vi "WAM_Datalog Parser.vi"() -> ()   [LabVIEW 2018]
uses:
  <vilib>/Utility/file.llb/Write Delimited Spreadsheet (DBL).vi
  <vilib>/Utility/file.llb/Read Delimited Spreadsheet (string).vi
  <vilib>/Utility/file.llb/Write Delimited Spreadsheet (string).vi
panel:
  out "Test Efficiency":string
  out "Fails Retested -Pass":i32
  out "Array":string[](array[string])
  out "pass_check-fails":string[](array[string])
  out "fails_check-pass":string[](array[string])
  out "Data 2":string[][](array[string])
  out "SN Search Result":string[][](array[string])
  in  "SN SEARCH":string
  out "tmp_path":path
  out "filenames":string[](array[string])
  out "Status":string
  out "Fails Repeated":i32
  out "Passes Repeated":i32
  out "#OfUnits_Adj":i32
  out "Total SN's Tested":i32
  out "#Passes_Adj":i32
  out "Pass Stats":cluster{"times":i32, "Word":string}[](array[cluster])
  out "Pass_sn":string[](array[string])
  out "Fails_Adj":i32
  out "No Of Words":i32
  out "Fail Stats":cluster{"times":i32, "Word":string}[](array[cluster])
  out "Fails_sn":string[](array[string])
  out "status":bool
  out "Message":string
  out "x > y?":bool
  in  "Get All Data(t)":bool
  out "Yield %":string
  out "Tested_Adj":i32
  out "End Date":string
  in  "Stop":timestamp
  out "Incompletes":string[][](array[string])
  out "# of Incompletes":i32
  in  "Use Today(t)":bool
  in  "Start":timestamp
  out "Fails":string[][](array[string])
  out "#Fails":i32
  out "Passed":string[][](array[string])
  out "#Passes":i32
  out "#of Tests":i32
  out "Tested  Data":string[][](array[string])
  out "Current Time":string
  out "Start Date":string
  out "Header":string[](array[string])
  out "Data":string[][](array[string])
  # "C:\\RageATE Results\\REV-C_TETRA_RX-PROD\\2_27_2023\\REV-C_TETRA_RX-PROD_SN_WAM-000422_2248_022723-094211.csv"
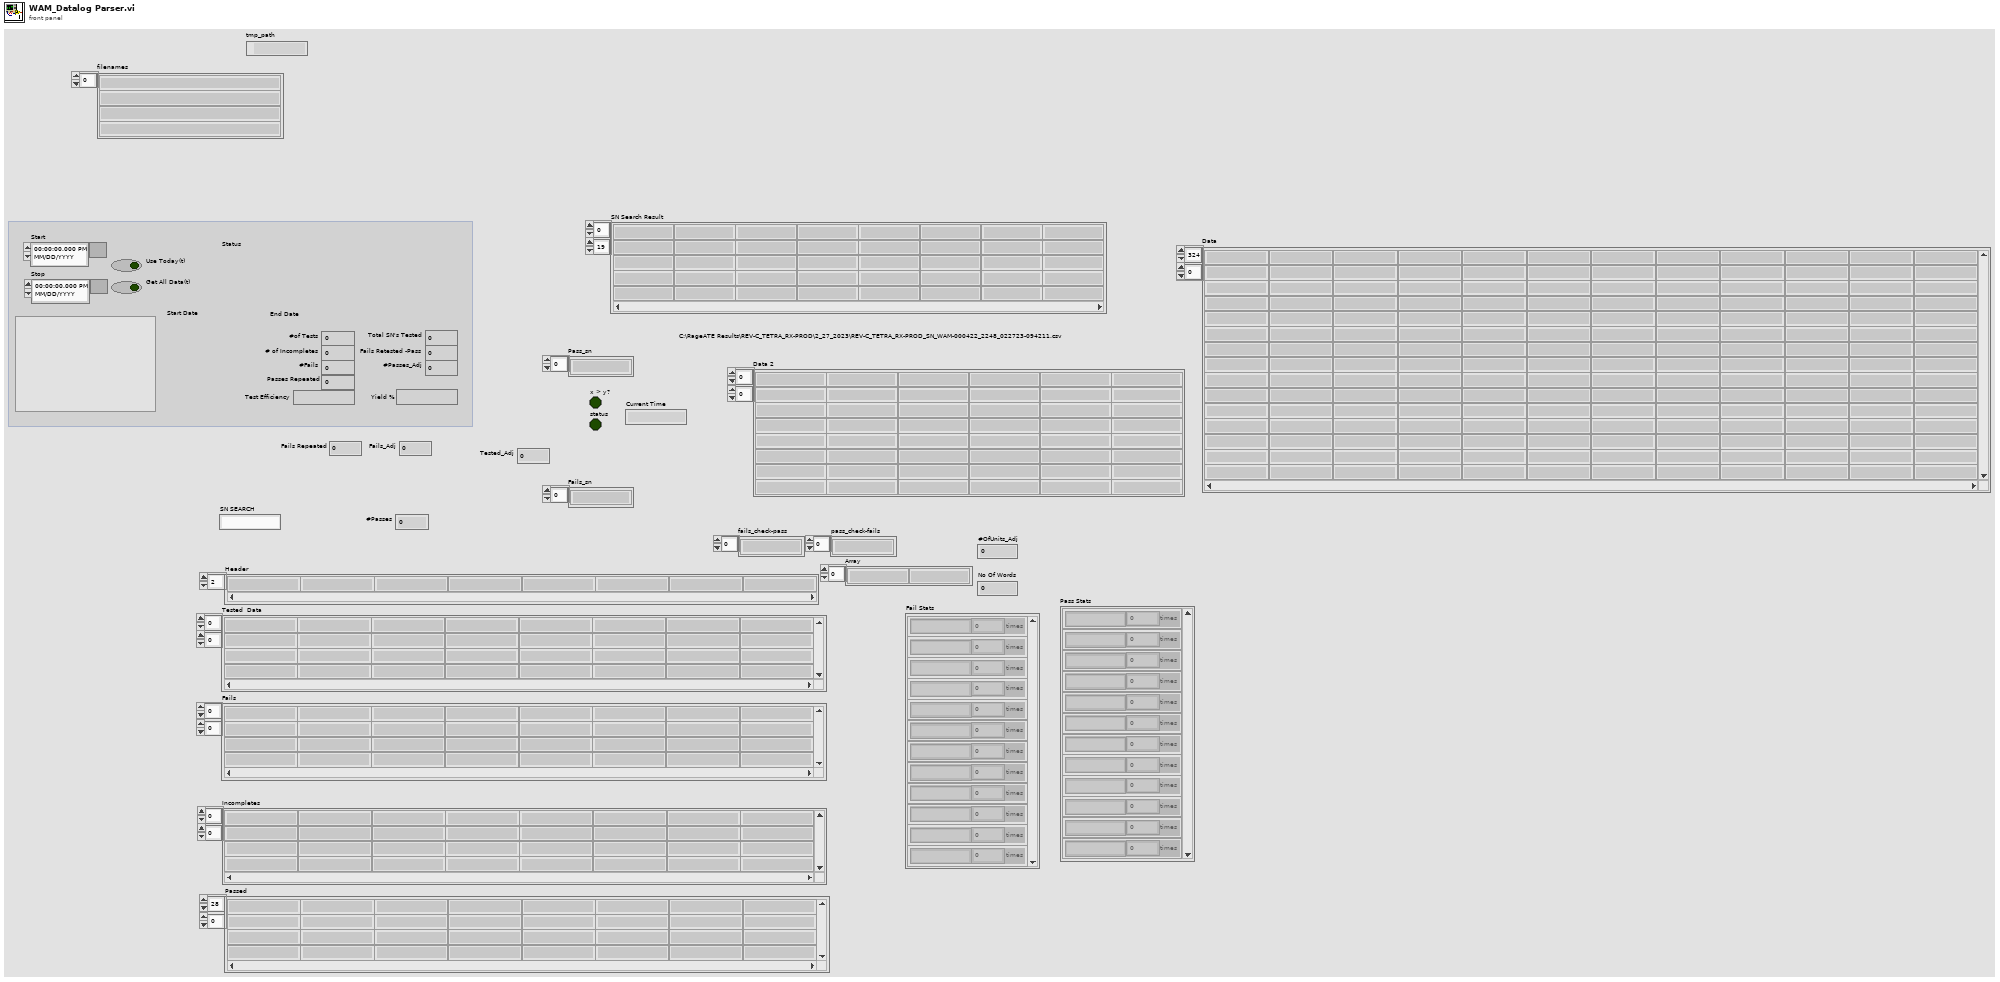
[diagram p1: front panel]
types:
  T1 = typedef "LVDateTimeRec.ctl" = cluster{"fractional second":dbl, "second":i32, "minute":i32, "hour":i32, "day of month":i32, "month":i32, "year":i32, "day of week":i32, "day of year":i32, "DST":i32}
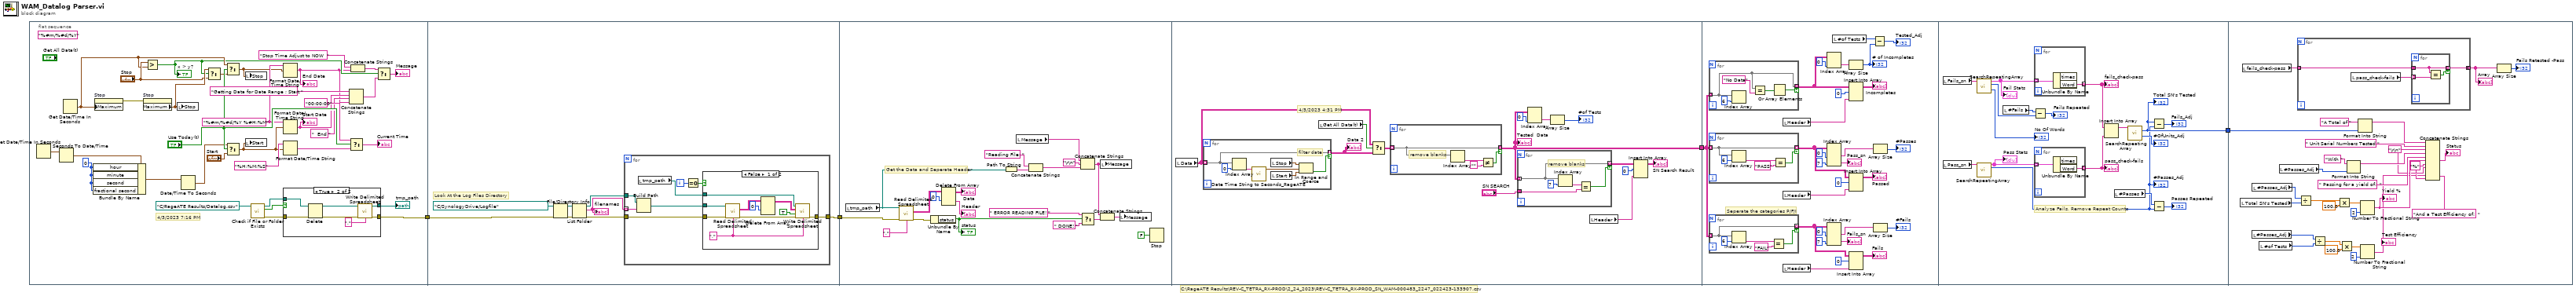
[diagram p0: block diagram]
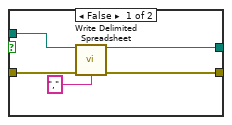
[diagram p2: hidden frame]
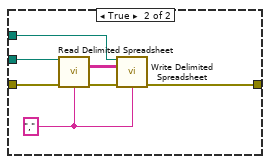
[diagram p3: hidden frame]
diagram:
  # "C:\\RageATE Results\\REV-C_TETRA_RX-PROD\\2_24_2023\\REV-C_TETRA_RX-PROD_SN_WAM-000483_2247_022423-133907.csv"
  n1 = flat-sequence {
    tunnel: [w13] -> w2
    tunnel: w2 -> [w53]
    tunnel: [w51] -> w1
    tunnel: w1 -> [w84]
    tunnel: [w104] -> w4
    tunnel: w4 -> [w160]
    tunnel: [w179] -> w3
    tunnel: w3 -> [w218]
    frame #0 {
      w7 = 0 ("hour")
      (unwired) "%#m/%#d/%Y" ("time format string (%c)")
      w12 = "%#m/%#d/%Y %#H:%M" ("time format string (%c)")
      # "4/3/2023 7:16 PM"
      n2 = Get Date/Time In Seconds() -> (seconds since 1Jan1904=w9:timestamp)
      n3 = Seconds To Date/Time(time stamp (now)=w9) -> (date time rec=w8:T1)  [unwired: 1 in]
      n4 = Get Date/Time In Seconds() -> (seconds since 1Jan1904=w28:timestamp)
      n5 = Bundle By Name(cluster=w8, "hour"=w7, "minute"=w7, "second"=w7, "fractional second"=w7) -> (w6:T1)
      n6 = property on="Stop" class="AbsTime (strict)"("Maximum"=w28) -> (error out=w32:errorcluster)  [unwired: 2 in, 1 out]
      n7 = property on="Stop" class="AbsTime (strict)"(error in=w32) -> ("Maximum"=w30:timestamp)  [unwired: 1 in, 2 out]
      n8 = Greater?(x="Stop", y=w28) -> (0:w27:bool)
      "x > y?" <- w27
      n9 = local write "Stop"(w30) -> ()
      n10 = Date/Time To Seconds(2:w6) -> (0:w5:timestamp)  [unwired: 1 in]
      n11 = Select(t=w30, s=w27, f="Stop") -> (s? t:f=w31:timestamp)
      n12 = Select(t=w28, s="Use Today(t)", f=w31) -> (s? t:f=w10:timestamp)
      n13 = Select(t=w5, s="Use Today(t)", f="Start") -> (s? t:f=w11:timestamp)
      n14 = local write "Stop"(w10) -> ()
      n15 = local write "Start"(w11) -> ()
      n16 = call <vilib>:"Check if File or Folder Exists.vi"("path"=path "C:/RageATE Results/Datalog.csv") -> ("error out"=w15:errorcluster, "file or folder exists?"=w17:bool, "dup path"=w16:path)  [unwired: 8 in]
      n17 = Format Date/Time String(time format string (%c)=w12, seconds (now)=w10) -> (date/time string=w20:string)  [unwired: 1 in]
      "End Date" <- w20
      n18 = Format Date/Time String(time format string (%c)=w12, seconds (now)=w11) -> (date/time string=w22:string)  [unwired: 1 in]
      "Start Date" <- w22
      n19 = Format Date/Time String(time format string (%c)="%H:%M:%S", seconds (now)=w11) -> (date/time string=w36:string)  [unwired: 1 in]
      n20 = case shown="True" w17 {
        tunnel: w16 -> [w42 w50]
        tunnel: w15 -> [w43 w49]
        tunnel: [w41 w46] -> w14
        tunnel: [w39 w44] -> w13
        frame False {
          n21 = call-poly <vilib>:"Write Delimited Spreadsheet.vi"("file path (dialog if empty)"=w42, "error in (no error)"=w43, "delimiter (\\t)"="," ("delimiter (\\t)")) -> ("new file path (Not A Path if cancelled)"=w41:path, "error out"=w39:errorcluster)  [unwired: 11 in]
        }
        frame True {
          n22 = Delete(path (use dialog)=w50, error in=w49) -> (deleted path=w48:path, error out=w47:errorcluster)  [unwired: 3 in, 1 out]
          n23 = call-poly <vilib>:"Write Delimited Spreadsheet.vi"("file path (dialog if empty)"=w48, "error in (no error)"=w47, "delimiter (\\t)"="," ("delimiter (\\t)")) -> ("new file path (Not A Path if cancelled)"=w46:path, "error out"=w44:errorcluster)  [unwired: 11 in]
        }
      }
      "tmp_path" <- w14
      n24 = Concatenate Strings("Getting Data for Date Range ; Start " ("string"), w22, "  End " ("string"), w20) -> (w19:string)
      n25 = Select(t="00:00:00", s="Use Today(t)", f=w36) -> (s? t:f=→"Current Time":string)
      n26 = Concatenate Strings("Stop Time Adjust to NOW  ", w20) -> (w24:string)
      n27 = Select(t=w24, s=w27, f=w19) -> (s? t:f=→"Message":string)
    }
    frame #1 {
      # "Look At the Log Files Directory"
      n28 = File/Directory Info(path=path "C:/SynologyDrive/Logfile" ("file path (dialog if empty)"), error in=w53) -> (path out=w57:path, error out=w56:errorcluster)  [unwired: 5 out]
      n29 = List Folder(path=w57, error in=w56) -> (path out=w55:path, filenames=w54:string[], error out=w52:errorcluster)  [unwired: 2 in, 1 out]
      "filenames" <- w54
      n30 = for {
        tunnel: w55 -> [w66]
        tunnel: w54 -> [w65] mode=indexing
        tunnel: w52 -> [w60]
        tunnel: [w59] -> w51
        i -> [w64]
        n31 = Build Path(base path=w66, name or relative path=w65) -> (appended path=w61:path)
        n32 = local read "tmp_path"() -> (w62:path)
        n33 = Equal To 0?(x=w64) -> (x = 0?=w63:bool)
        n34 = case shown="False" w63 {
          tunnel: w62 -> [w76 w83]
          tunnel: w61 -> [w75 w81]
          tunnel: w60 -> [w69 w77]
          tunnel: [w67 w79] -> w59
          frame False {
            w71 = "," ("delimiter (\\t)")
            n35 = call-poly <vilib>:"Read Delimited Spreadsheet.vi"("file path (dialog if empty)"=w75, "error in (no error)"=w69, "delimiter (\\t)"=w71) -> ("all rows"=w74:string[][], "error out"=w68:errorcluster)  [unwired: 7 in, 4 out]
            n36 = Delete From Array(array=w74, index (row)=0) -> (array with subset deleted=w73:string[][])  [unwired: 2 in, 1 out]
            n37 = call-poly <vilib>:"Write Delimited Spreadsheet.vi"("file path (dialog if empty)"=w76, "2D data"=w73, "append to file? (new file:F)"=TRUE, "error in (no error)"=w68, "delimiter (\\t)"=w71) -> ("error out"=w67:errorcluster)  [unwired: 9 in, 1 out]
          }
          frame True {
            w80 = "," ("delimiter (\\t)")
            n38 = call-poly <vilib>:"Read Delimited Spreadsheet.vi"("file path (dialog if empty)"=w81, "error in (no error)"=w77, "delimiter (\\t)"=w80) -> ("all rows"=w82:string[][], "error out"=w78:errorcluster)  [unwired: 7 in, 4 out]
            n39 = call-poly <vilib>:"Write Delimited Spreadsheet.vi"("file path (dialog if empty)"=w83, "2D data"=w82, "error in (no error)"=w78, "delimiter (\\t)"=w80) -> ("error out"=w79:errorcluster)  [unwired: 10 in, 1 out]
          }
        }
      }
    }
    frame #2 {
      # "Get the Data and Seperate Header"
      n40 = local read "tmp_path"() -> (w85:path)
      n41 = call-poly <vilib>:"Read Delimited Spreadsheet.vi"("file path (dialog if empty)"=w85, "error in (no error)"=w84, "delimiter (\\t)"="," ("delimiter (\\t)")) -> ("all rows"=w102:string[][], "error out"=w93:errorcluster)  [unwired: 7 in, 4 out]
      n42 = Unbundle By Name(w93) -> ("status"=w92:bool)
      "status" <- w92
      n43 = Delete From Array(array=w102, index (row)=0) -> (deleted portion=→"Header":string[], array with subset deleted=→"Data":string[][])  [unwired: 2 in]
      n44 = Path To String(path=w85) -> (string=w95:string)
      n45 = local read "Message"() -> (w98:string)
      n46 = Concatenate Strings("Reading File: ", w95) -> (w94:string)
      n47 = Concatenate Strings(w98, "\r\n", w94) -> (w91:string)
      n48 = Select(t=" ERROR READING FILE! ", s=w92, f=" DONE! ") -> (s? t:f=w88:string)
      n49 = local write "Message"(w91) -> ()
      n50 = Concatenate Strings(w91, w88) -> (w87:string)
      n51 = local write "Message"(w87) -> ()
      n52 = Stop(stop? (T)=FALSE) -> ()
    }
    frame #3 {
      # "4/3/2023 4:31 PM"
      n53 = local read "Data"() -> (w115:string[][])
      n54 = for {
        tunnel: w115 -> [w128] mode=indexing
        tunnel: [w128] -> w114 mode=indexing if=w132
        # "filter date"
        n55 = Index Array(array=w128, index=0) -> (element=w127:string)
        n56 = call "Date Time String to Seconds_RageATE.vi"("Time/date(str)in"=w127) -> ("Timestamp from Date/Time String"=w126:timestamp)  [unwired: 8 in, 2 out]
        n57 = local read "Stop"() -> (w129:timestamp)
        n58 = local read "Start"() -> (w130:timestamp)
        n59 = In Range and Coerce(upper limit=w129, x=w126, lower limit=w130) -> (In Range?=w132:bool)  [unwired: 1 out]
      }
      "Data 2" <- w114
      n60 = local read "Get All Data(t)"() -> (w113:bool)
      n61 = Select(t=w115, s=w113, f=w114) -> (s? t:f=w116:string[][])
      n62 = for {
        tunnel: [w123] -> w104 mode=indexing if=w125
        tunnel: w116 -> [w123] mode=indexing
        # "remove blanks"
        n63 = Index Array(array=w123) -> (element=w122:string)  [unwired: 1 in]
        n64 = Not Equal?(x=w122, y="") -> (x != y?=w125:bool)
      }
      "Tested  Data" <- w104
      n65 = for {
        tunnel: [w120] -> w108 mode=indexing if=w121
        tunnel: w104 -> [w120] mode=indexing
        tunnel: "SN SEARCH" -> [w117]
        # "remove blanks"
        n66 = Index Array(array=w120, index=7) -> (element=w119:string)
        n67 = Equal?(x=w119, y=w117) -> (x = y?=w121:bool)
      }
      n68 = Index Array(array=w104, index (col)=0 ("disabled index (col)")) -> (element=w111:string[])  [unwired: 1 in]
      n69 = Array Size(array=w111) -> (size(s)=→"#of Tests":i32)
      n70 = local read "Header"() -> (w106:string[])
      n71 = Insert Into Array(array=w108, index (row)=0, new element=w106) -> (→"SN Search Result":string[][])  [unwired: 1 in]
    }
    frame #4 {
      # "Seperate the categories P/F/I"
      n72 = for {
        tunnel: [w163] -> w148 mode=indexing if=w161
        tunnel: w160 -> [w163] mode=indexing
        n73 = Index Array(array=w163, index=6) -> ()  [unwired: 1 out]
        n74 = Equal?(x=w163, y="No Data") -> (x = y?=w162:bool[])
        n75 = Or Array Elements(Boolean array=w162) -> (logical OR=w161:bool)
      }
      n76 = for {
        tunnel: [w174] -> w145 mode=indexing if=w175
        tunnel: w160 -> [w174] mode=indexing
        n77 = Index Array(array=w174, index=6) -> (element=w173:string)
        n78 = Equal?(x=w173, y="PASS") -> (x = y?=w175:bool)
      }
      n79 = for {
        tunnel: [w169] -> w140 mode=indexing if=w170
        tunnel: w160 -> [w169] mode=indexing
        n80 = Index Array(array=w169, index=6) -> (element=w168:string)
        n81 = Equal?(x=w168, y="FAIL") -> (x = y?=w170:bool)
      }
      n82 = local read "Header"() -> (w153:string[])
      n83 = local read "Header"() -> (w157:string[])
      n84 = local read "Header"() -> (w154:string[])
      n85 = Index Array(array=w148, index (col)=0 ("disabled index (col)")) -> (element=w150:string[])  [unwired: 1 in]
      n86 = Index Array(array=w145, index (col) #1=0 ("disabled index (col)"), index (col) #2=7 ("index (col)")) -> (element #1=w159:string[], element #2=→"Pass_sn":string[])  [unwired: 2 in]
      n87 = Index Array(array=w140, index (col) #1=0 ("disabled index (col)"), index (col) #2=7 ("index (col)")) -> (element #1=w143:string[], element #2=→"Fails_sn":string[])  [unwired: 2 in]
      n88 = local read "#of Tests"() -> (w138:i32)
      n89 = Array Size(array=w150) -> (size(s)=w139:i32)
      "# of Incompletes" <- w139
      n90 = Insert Into Array(array=w148, index (row)=0, new element=w153) -> (→"Incompletes":string[][])  [unwired: 1 in]
      n91 = Insert Into Array(array=w145, index (row)=0, new element=w157) -> (→"Passed":string[][])  [unwired: 1 in]
      n92 = Insert Into Array(array=w140, index (row)=0, new element=w154) -> (→"Fails":string[][])  [unwired: 1 in]
      n93 = Subtract(x=w138, y=w139) -> (x-y=→"Tested_Adj":i32)
      n94 = Array Size(array=w159) -> (size(s)=→"#Passes":i32)
      n95 = Array Size(array=w143) -> (size(s)=→"#Fails":i32)
    }
    frame #5 {
      # "Analyze Fails, Remove Repeat Counts"
      n96 = local read "Fails_sn"() -> (w176:string[])
      n97 = local read "Pass_sn"() -> (w192:string[])
      n98 = call "SearchRepeatingArray.vi"("Input(ary)"=w176) -> ("Statistics"=w191:cluster{"times":i32, "Word":string}[], "No Of Unique Words"=w182:i32, "No Of Words"=→"No Of Words":i32)  [unwired: 11 in, 1 out]
      "Fail Stats" <- w191
      n99 = call "SearchRepeatingArray.vi"("Input(ary)"=w192) -> ("Statistics"=w190:cluster{"times":i32, "Word":string}[], "No Of Unique Words"=w178:i32)  [unwired: 11 in, 2 out]
      "Pass Stats" <- w190
      "#Passes_Adj" <- w178
      n100 = local read "#Fails"() -> (w181:i32)
      n101 = Subtract(x=w181, y=w182) -> (x-y=→"Fails Repeated":i32)
      n102 = for {
        tunnel: w191 -> [w196] mode=indexing
        tunnel: [w195] -> w188 mode=indexing
        n103 = Unbundle By Name(w196) -> ("Word"=w195:string)  [unwired: 1 out]
      }
      "fails_check-pass" <- w188
      n104 = for {
        tunnel: w190 -> [w194] mode=indexing
        tunnel: [w193] -> w177 mode=indexing
        n105 = Unbundle By Name(w194) -> ("Word"=w193:string)  [unwired: 1 out]
      }
      "pass_check-fails" <- w177
      n106 = Insert Into Array(array=w188, new element=w177) -> (w187:string[])  [unwired: 1 in]
      n107 = local read "#Passes"() -> (w184:i32)
      n108 = call "SearchRepeatingArray.vi"("Input(ary)"=w187) -> ("No Of Unique Words"=w179:i32, "No Of Words"=→"#OfUnits_Adj":i32)  [unwired: 11 in, 2 out]
      "Total SN's Tested" <- w179
      n109 = Subtract(x=w179, y=w178) -> (x-y=→"Fails_Adj":i32)
      n110 = Subtract(x=w184, y=w178) -> (x-y=→"Passes Repeated":i32)
    }
    frame #6 {
      w200 = "%" ("string")
      w202 = "\r\n"
      n111 = local read "Total SN's Tested"() -> (w222:i32)
      n112 = local read "fails_check-pass"() -> (w210:string[])
      n113 = local read "#Passes_Adj"() -> (w207:i32)
      n114 = local read "#Passes_Adj"() -> (w223:i32)
      n115 = local read "#of Tests"() -> (w206:i32)
      n116 = local read "#Passes_Adj"() -> (w214:i32)
      n117 = for {
        tunnel: w210 -> [w228] mode=indexing
        tunnel: [w226] -> w209 mode=concatenating
        n118 = local read "pass_check-fails"() -> (w227:string[])
        n119 = for {
          tunnel: w228 -> [w230]
          tunnel: w227 -> [w231] mode=indexing
          tunnel: [w230] -> w226 mode=indexing if=w229
          n120 = Equal?(x=w230, y=w231) -> (x = y?=w229:bool)
        }
      }
      "Array" <- w209
      n121 = Divide(x=w223, y=w222) -> (x/y=w221:dbl)
      n122 = Divide(x=w207, y=w206) -> (x/y=w204:dbl)
      n123 = Multiply(x=w221, y=100.0) -> (x*y=w224:dbl)
      n124 = Multiply(x=w204, y=100.0) -> (x*y=w203:dbl)
      n125 = Format Into String(initial string="With ", w214) -> (resulting string=w213:string)  [unwired: 2 in, 1 out]
      n126 = Format Into String(initial string="A Total of ", w218) -> (resulting string=w217:string)  [unwired: 2 in, 1 out]
      n127 = Number To Fractional String(number=w203, precision (6)=i16 2) -> (F-format string=w199:string)  [unwired: 2 in]
      "Test Efficiency" <- w199
      n128 = Number To Fractional String(number=w224, precision (6)=i16 2) -> (F-format string=w211:string)  [unwired: 2 in]
      "Yield %" <- w211
      n129 = Concatenate Strings(w217, " Unit Serial Numbers Tested " ("string"), w202, w213, " Passing for a yield of:  " ("string"), w211, w200, w202, "And a Test Efficiency of:  " ("string"), w199, w200) -> (→"Status":string)
      n130 = Array Size(array=w209) -> (size(s)=→"Fails Retested -Pass":i32)
    }
  }
